vi "Set_Bandwidth_DHPCA-100.vi"(3 "error in":errorcluster, 4 "Status":i32, 5 "Bandwidth":enum16{"Full Bandwidth", "10 MHz", "1MHz"}(ring), 6 "index":i32) -> (0 "error out":errorcluster, 1 "Status_out":i32, 2 "index_out":i32)   [LabVIEW 2010, in "FEMTO_LUCI-10.lvlib"]
uses:
  <userlib>/FEMTO/FEMTO_LUCI-10.lvlib
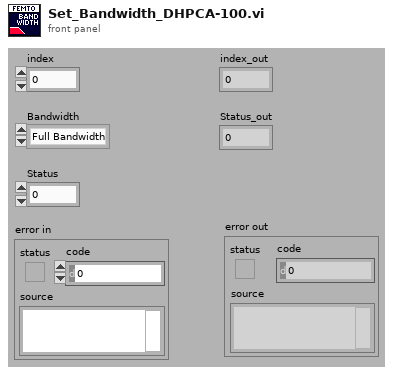
[diagram p1: front panel]
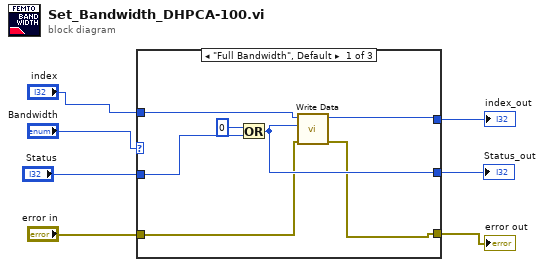
[diagram p0: block diagram]
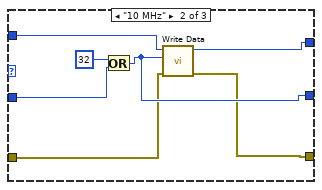
[diagram p2: hidden frame]
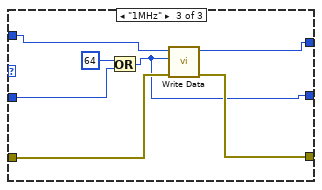
[diagram p3: hidden frame]
diagram:
  n1 = case shown="\"Full Bandwidth\", Default" "Bandwidth" {
    tunnel: [w11 w21 w22] -> w7
    tunnel: "Status" -> [w10 w20 w25]
    tunnel: [w8 w19 w23] -> w5
    tunnel: "error in" -> [w9 w18 w24]
    tunnel: [w12 w17 w26] -> w3
    tunnel: "index" -> [w13 w16 w27]
    frame "Full Bandwidth", Default {
      n2 = Or(x=0 ("data_low"), y=w10) -> (x .or. y?=w11:i32)
      n3 = call <userlib>:"Write Data.vi"("error in (no error)"=w9, "data_low"=w11, "index"=w13) -> ("error out"=w8:errorcluster, "index_out"=w12:i32)  [unwired: 1 in, 6 out]
    }
    frame "10 MHz" {
      n4 = Or(x=32 ("data_low"), y=w20) -> (x .or. y?=w21:i32)
      n5 = call <userlib>:"Write Data.vi"("error in (no error)"=w18, "data_low"=w21, "index"=w16) -> ("error out"=w19:errorcluster, "index_out"=w17:i32)  [unwired: 1 in, 6 out]
    }
    frame "1MHz" {
      n6 = Or(x=64 ("data_low"), y=w25) -> (x .or. y?=w22:i32)
      n7 = call <userlib>:"Write Data.vi"("error in (no error)"=w24, "data_low"=w22, "index"=w27) -> ("error out"=w23:errorcluster, "index_out"=w26:i32)  [unwired: 1 in, 6 out]
    }
  }
  "index_out" <- w3
  "error out" <- w5
  "Status_out" <- w7
